vi "teleop.vi"() -> ()   [LabVIEW 2012, in "Robot Green.lvrbt"]
uses:
  Robot Green.lvrbt
  <vilib>/NXT/Hardware/Plugins/Tetrix DC Motor/TetrixDCMotorAddress.ctl
  <vilib>/NXT/Hardware/Plugins/Tetrix 180 deg Servo/Tetrix180ServoAddress.ctl
  <vilib>/FTC/FTC Read Controller Packet.vi
  <vilib>/FTC/FTC Calculate Drive Power - Tank.vi
  <vilib>/FTC/FTC Read Button States.vi
  <vilib>/NXT/NXTIO Xnodes/NXTIONodeSubVIs/TETRIX IO Move DC Motors.vi
  <vilib>/NXT/NXTIO Xnodes/NXTIONodeSubVIs/TETRIX IO Move Servos.vi
  <vilib>/NXT/NXTIO Xnodes/NXTIONodeSubVIs/TETRIX IO Stop DC Motors.vi
  <vilib>/NXT/NXTIO Xnodes/NXTIONodeSubVIs/TETRIX IO Check Battery.vi
  <vilib>/NXT/NXTIO Xnodes/AddressXNode/NXTIOAddress.xnode
  <vilib>/NXT/Subs/LVHSConnector.ctl
  <vilib>/NXT/NXTIO Xnodes/NXTIOXNode/NXTIO.xnode
  <vilib>/NXT/LegoClasses/BrickReference/BrickReference.lvclass
panel:
  in  "Drive Power":i8=75 min=-100 max=100
  # "This VI was generated based on your configuration in the Remote Control Editor. You may modify the code as needed for your robot. To test this program for an FTC match, return to the Remote Control Editor, select the \"Run Program\" tab, and choose \"Teleop\"."
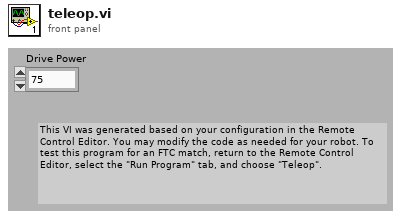
[diagram p1: front panel]
types:
  T1 = typedef "TetrixDCMotorAddress.ctl" = i32
  T2 = cluster{"TetrixDCMotor":T1, "TetrixDCMotor 2":T1}
  T3 = typedef "LVHSConnector.ctl" = refnum<class "BrickReference.lvclass">
  T4 = typedef "FTC ControllerState.ctl" = cluster{"Left X":i8, "Left Y":i8, "Right X":i8, "Right Y":i8, "Button Encoding 9-12":u8, "Button Encoding 1-8":u8, "POV":T5}
  T5 = typedef "FTC POVState.ctl" = i8
  T6 = typedef "FTC ButtonEventType.ctl" = enum16{"Pressed", "Released"}
  T7 = cluster{"Button ID":enum16{"None", "Button 1", "Button 2", "Button 3", "Button 4", "Button 5", "Button 6", "Button 7", "Button 8", "Button 9", "Button 10", "Button 11", "Button 12", "POV Up", "POV Up Right", "POV Right", "POV Down Right", "POV Down", "POV Down Left", "POV Left", "POV Up Left"}, "Event Type":T6}[]
  T8 = enum16{"None", "Button 1", "Button 2", "Button 3", "Button 4", "Button 5", "Button 6", "Button 7", "Button 8", "Button 9", "Button 10", "Button 11", "Button 12", "POV Up", "POV Up Right", "POV Right", "POV Down Right", "POV Down", "POV Down Left", "POV Left", "POV Up Left"}
  T9 = typedef "Tetrix180ServoAddress.ctl" = i32
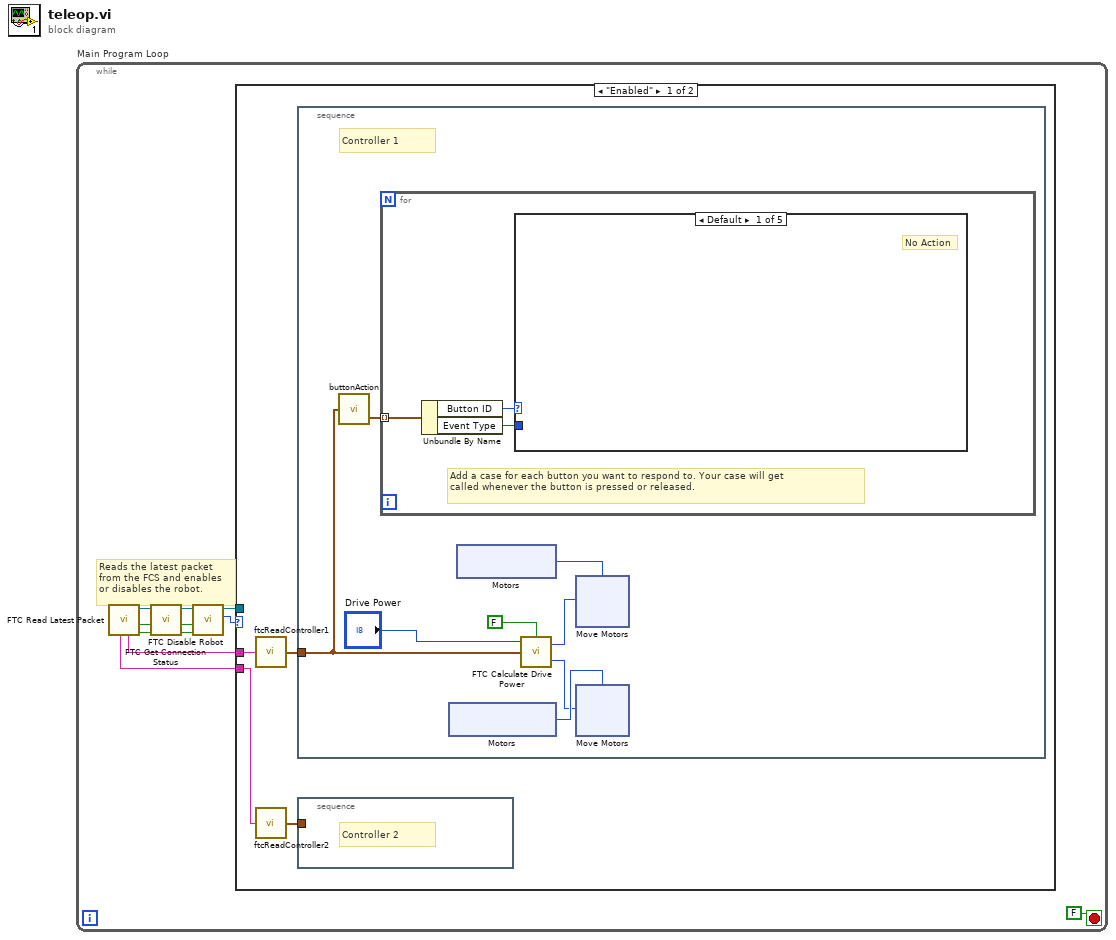
[diagram p0: block diagram]
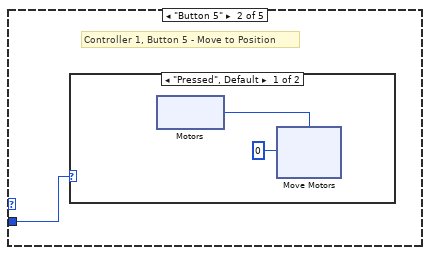
[diagram p2: hidden frame]
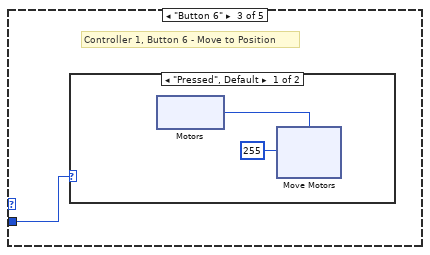
[diagram p4: hidden frame]
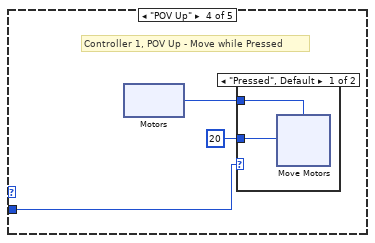
[diagram p6: hidden frame]
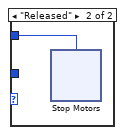
[diagram p7: hidden frame]
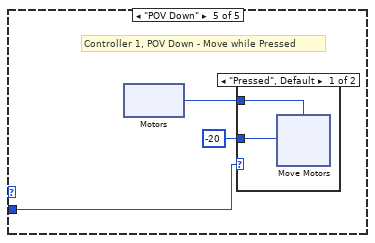
[diagram p8: hidden frame]
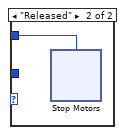
[diagram p9: hidden frame]
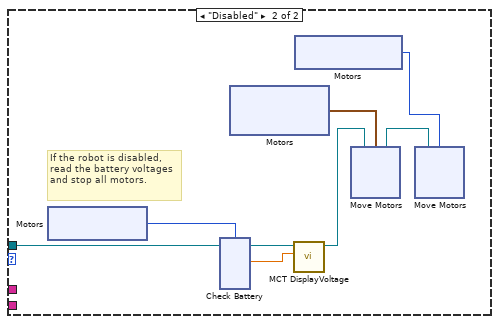
[diagram p10: hidden frame]
diagram:
  n1 = while "Main Program Loop" {
    stop <- FALSE stop-if-true
    # "Reads the latest packet\nfrom the FCS and enables\nor disables the robot."
    n2 = call <vilib>:"FTC Read Latest Packet.vi"() -> ("Packet Received?"=w8:bool, "Stopped?"=w5:bool, "NXT/EV3"=w7:T3, "Controller 1"=w10:string, "Controller 2"=w9:string)  [unwired: 6 in, 1 out]
    n3 = call <vilib>:"FTC Get Connection Status.vi"("Packet Received?"=w8, "Stopped?"=w5, "NXT/EV3"=w7) -> ("Online?"=w2:bool, "Stopped?"=w3:bool, "NXT/EV3"=w4:T3)  [unwired: 5 in]
    n4 = call <vilib>:"FTC Disable Robot.vi"("Online?"=w2, "Stopped?"=w3, "NXT/EV3"=w4) -> ("Enabled?"=w6:enum16{"Disabled", "Enabled"}, "NXT/EV3"=w1:T3)  [unwired: 3 in]
    n5 = case "disableCase" shown="\"Enabled\"" w6 {
      tunnel: w10 -> [w15 _]
      tunnel: w9 -> [w14 _]
      tunnel: w1 -> [_ w110]
      frame "Enabled" {
        n6 = call "ftcReadController1"("Packet"=w15) -> ("Controller State"=w13:T4)  [unwired: 4 in]
        n7 = call "ftcReadController2"("Packet"=w14) -> ("Controller State"=w12:T4)  [unwired: 4 in]
        n8 = stacked-sequence "controller1Actions" {
          tunnel: w13 -> [w22]
          frame #0 {
            # "Controller 1"
            n9 = call "buttonAction"("Controller State"=w22) -> ("Button Events"=w23:T7)  [unwired: 2 in, 1 out]
            n10 = for "buttonAction" {
              tunnel: w23 -> [w40] mode=indexing
              # "Add a case for each button you want to respond to. Your case will get \ncalled whenever the button is pressed or released."
              n11 = Unbundle By Name(w40) -> ("Button ID"=w42:T8, "Event Type"=w41:T6)
              n12 = case "EventCase1" shown="Default" w42 {
                tunnel: w41 -> [_ w43 w54 w67 w86]
                frame Default {
                  # "No Action"
                }
                frame "Button 5" {
                  # "Controller 1, Button 5 - Move to Position"
                  n13 = case shown="\"Pressed\", Default" w43 {
                    frame "Pressed", Default {
                      n14 = xnode "Motors"() -> ("Motor"=w45:T9)
                      n15 = xnode "Move Motors"("Position 1"=0, "Motors"=w45) -> ()  [unwired: 1 in, 1 out]
                    }
                    frame "Released" {
                    }
                  }
                }
                frame "Button 6" {
                  # "Controller 1, Button 6 - Move to Position"
                  n16 = case shown="\"Pressed\", Default" w54 {
                    frame "Pressed", Default {
                      n17 = xnode "Motors"() -> ("Motor"=w56:T9)
                      n18 = xnode "Move Motors"("Position 1"=255, "Motors"=w56) -> ()  [unwired: 1 in, 1 out]
                    }
                    frame "Released" {
                    }
                  }
                }
                frame "POV Up" {
                  # "Controller 1, POV Up - Move while Pressed"
                  n19 = xnode ("Motors")() -> ("Motor"=w65:T1)
                  n20 = case shown="\"Pressed\", Default" w67 {
                    tunnel: 20 ("Power (75)") -> [w70 _]
                    tunnel: w65 -> [w69 w78]
                    frame "Pressed", Default {
                      n21 = xnode "Move Motors"("Power/Speed 1"=w70, "Motors"=w69) -> ()  [unwired: 1 in, 1 out]
                    }
                    frame "Released" {
                      n22 = xnode "Stop Motors"("Motors"=w78) -> ()  [unwired: 1 in, 1 out]
                    }
                  }
                }
                frame "POV Down" {
                  # "Controller 1, POV Down - Move while Pressed"
                  n23 = xnode ("Motors")() -> ("Motor"=w84:T1)
                  n24 = case shown="\"Pressed\", Default" w86 {
                    tunnel: -20 ("Power (75)") -> [w89 _]
                    tunnel: w84 -> [w88 w97]
                    frame "Pressed", Default {
                      n25 = xnode "Move Motors"("Power/Speed 1"=w89, "Motors"=w88) -> ()  [unwired: 1 in, 1 out]
                    }
                    frame "Released" {
                      n26 = xnode "Stop Motors"("Motors"=w97) -> ()  [unwired: 1 in, 1 out]
                    }
                  }
                }
              }
            }
            n27 = xnode "Motors"() -> ("Motor"=w19:T1)
            n28 = xnode "Motors"() -> ("Motor"=w17:T1)
            n29 = call-poly <vilib>:"FTC Calculate Drive Power.vi"("Reverse"=FALSE, "Controller State"=w22, "Power Level (50)"="Drive Power") -> ("Right Motor Power"=w18:i8, "Left Motor Power"=w16:i8)  [unwired: 1 in]
            n30 = xnode "Move Motors"("Power/Speed 1"=w16, "Motors"=w17) -> ()  [unwired: 1 in, 1 out]
            n31 = xnode "Move Motors"("Power/Speed 1"=w18, "Motors"=w19) -> ()  [unwired: 1 in, 1 out]
          }
        }
        n32 = stacked-sequence "controller2Actions" {
          tunnel: w12 -> [_]
          frame #0 {
            # "Controller 2"
          }
        }
      }
      frame "Disabled" {
        # "If the robot is disabled, read the battery voltages and stop all motors."
        n33 = xnode ("Motors")() -> ("Motor"=w109:T1)
        n34 = xnode ("Check Battery")("Motors"=w109, "NXT/EV3"=w110) -> ("Voltage 1"=w108:sgl, "NXT/EV3"=w107:T3)
        n35 = xnode "Motors"() -> ("Motor"=w106:cluster{"TetrixDCMotor":T1, "TetrixDCMotor":T1})
        n36 = call <vilib>:"MCT DisplayVoltage.vi"("Motor Voltage"=w108, "NXT/EV3"=w107) -> ("NXT/EV3"=w105:T3)  [unwired: 9 in]
        n37 = xnode "Motors"() -> ("Motor"=w104:T1)
        n38 = xnode "Move Motors"("Motors"=w106, "NXT/EV3"=w105) -> ("NXT/EV3"=w103:T3)
        n39 = xnode "Move Motors"("Motors"=w104, "NXT/EV3"=w103) -> ()  [unwired: 1 out]
      }
    }
  }
